vi "Read rotator.vi"(8 "error in (no error)":errorcluster, 11 "ScienceTargetConfiguration in":refnum<class "ScienceTargetConfiguration.lvclass">) -> (0 "error out":errorcluster, 2 "Rotator.lvclass":refnum<class "Rotator.lvclass">, 3 "ScienceTargetConfiguration out":refnum<class "ScienceTargetConfiguration.lvclass">)   [LabVIEW 2022 SP3, in "TCSDataDefinitions.lvlib" / "TCSCommand.lvlib" / "TargetConfiguration.lvlib" / "ScienceTargetConfiguration.lvclass"]
uses:
  ScienceTargetConfiguration.lvclass
  Rotator/Rotator.lvclass
  ScienceTargetConfiguration.lvclass/ScienceTargetConfiguration.ctl
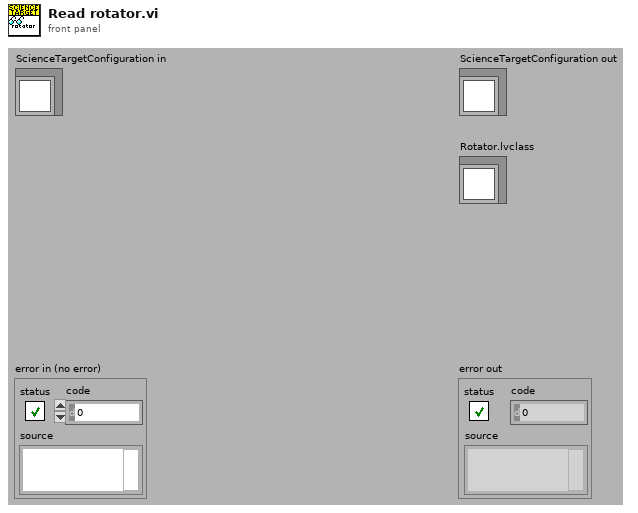
[diagram p1: front panel]
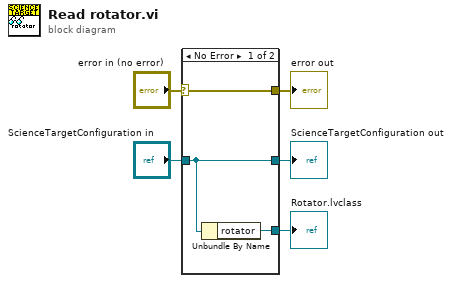
[diagram p0: block diagram]
diagram:
  n1 = case shown="No Error" "error in (no error)" {
    selector: "error in (no error)" -> [w8 w9]
    tunnel: [w8 w9] -> w4
    tunnel: [w7 w10] -> w2
    tunnel: "ScienceTargetConfiguration in" -> [w7 w10]
    tunnel: [w6 _] -> w1
    frame No Error {
      n2 = Unbundle By Name(w7) -> ("rotator"=w6:refnum<class "Rotator.lvclass">)
    }
    frame Error {
    }
  }
  "error out" <- w4
  "ScienceTargetConfiguration out" <- w2
  "Rotator.lvclass" <- w1
